vi "Actualizar Credito.vi"(8 "error in (no error)":errorcluster, 10 "Cluster":T1, 11 "USD Actor in":refnum<class "USD Actor.lvclass">) -> (0 "error out":errorcluster, 3 "USD Actor out":refnum<class "USD Actor.lvclass">)   [LabVIEW 2019, in "USD Actor.lvlib" / "USD Actor.lvclass"]
uses:
  USD Actor.lvclass
  C:/Program Files (x86)/National Instruments/LabVIEW 2019/vi.lib/ActorFramework/Actor/Actor.lvclass
  <vilib>/ActorFramework/Actor/Actor.lvclass/Actor.ctl
  USD Actor.lvclass/USD Actor.ctl
  UI Actor Messages/Actualiza Credito Msg/Actualiza Credito Msg.lvclass/Actualiza Credito Msg.ctl
  <vilib>/ActorFramework/Message Enqueuer/Message Enqueuer.lvclass/Message Enqueuer.ctl
  <vilib>/ActorFramework/Message Enqueuer/Enqueue.vi
  UI Actor Messages/Actualiza Credito Msg/Actualiza Credito Msg.lvclass
  C:/Program Files (x86)/National Instruments/LabVIEW 2019/vi.lib/ActorFramework/Message/Message.lvclass
  <vilib>/ActorFramework/Message Priority Queue/Priority Enqueue.vi
  <vilib>/ActorFramework/Actor/Actor.lvclass
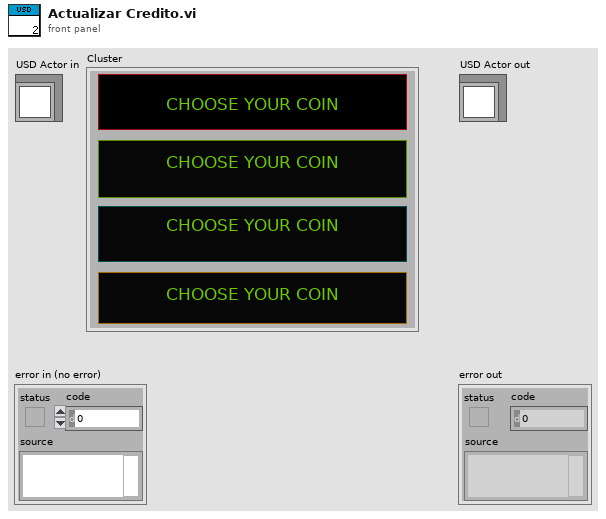
[diagram p1: front panel]
types:
  T1 = cluster{"COIN 1":bool, "COIN 2":bool, "COIN 3":bool, "COIN 4":bool}
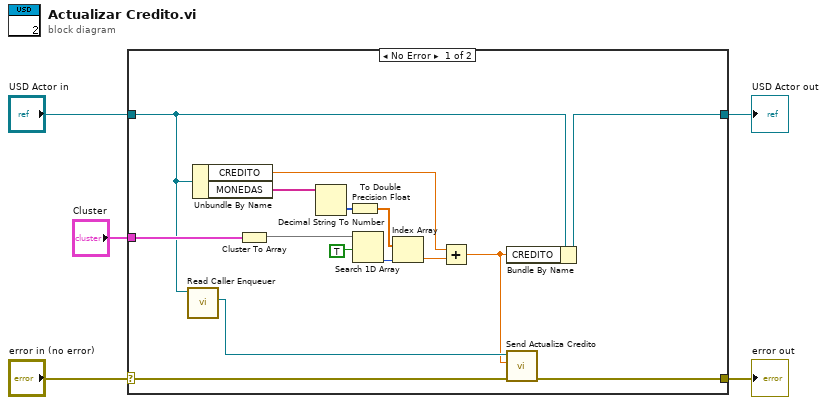
[diagram p0: block diagram]
diagram:
  n1 = case shown="No Error" "error in (no error)" {
    selector: "error in (no error)" -> [w8 w22]
    tunnel: [w7 w22] -> w2
    tunnel: [w15 w21] -> w3
    tunnel: "USD Actor in" -> [w10 w21]
    tunnel: "Cluster" -> [w12 _]
    frame No Error {
      n2 = call <vilib>:"Read Caller Enqueuer.vi"("Actor"=w10) -> ("Caller Enqueuer"=w9:refnum<class "Message Enqueuer.lvclass">)  [unwired: 10 in]
      n3 = Unbundle By Name(w10) -> ("CREDITO"=w11:dbl, "MONEDAS"=w18:string[])
      n4 = Cluster To Array(cluster=w12) -> (array=w13:bool[])
      n5 = Decimal String To Number(string=w18) -> (number=w17:i32[])  [unwired: 2 in, 1 out]
      n6 = To Double Precision Float(number=w17) -> (double precision float=w16:dbl[])
      n7 = Search 1D Array(1D array=w13, element=TRUE) -> (index of element=w19:i32)  [unwired: 1 in]
      n8 = Index Array(array=w16, index=w19) -> (element=w14:dbl)
      n9 = Add(x=w11, y=w14) -> (x+y=w6:dbl)
      n10 = Bundle By Name(cluster=w10, "CREDITO"=w6) -> (w15:refnum<class "USD Actor.lvclass">)
      n11 = call "Send Actualiza Credito.vi"("error in (no error)"=w8, "CREDITO ACTUAL"=w6, "Message Enqueuer"=w9) -> ("error out"=w7:errorcluster)  [unwired: 7 in, 1 out]
    }
    frame Error {
    }
  }
  "error out" <- w2
  "USD Actor out" <- w3
